vi "Send Next State.vi"(8 "error in (no error)":errorcluster, 9 "Data":variant, 10 "State":string, 11 "ExampleSimpleRootModel in":refnum<class "SimpleRootModel.lvclass">) -> (0 "error out":errorcluster, 3 "ExampleSimpleRootModel out":refnum<class "SimpleRootModel.lvclass">)   [LabVIEW 2018, in "MVAExamples.lvlib" / "SimpleRootModel.lvclass"]
uses:
  SimpleRootModel.lvclass
  <vilib>/ActorFramework/Actor/Actor.lvclass
  ExampleSimpleRootModel Messages/Execute State Msg/Execute State Msg.lvclass
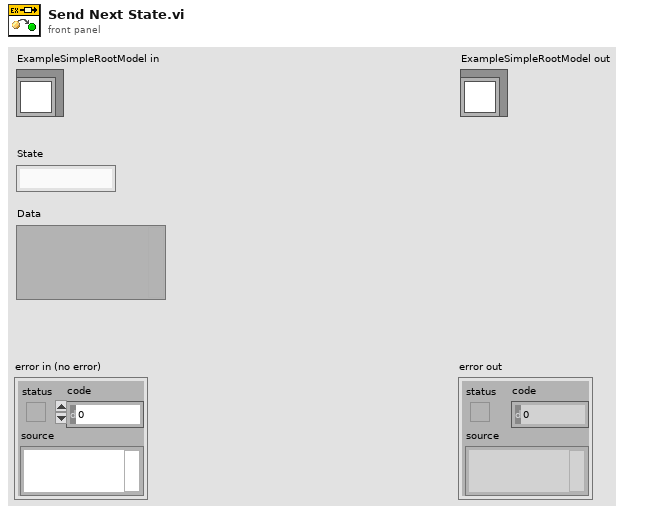
[diagram p1: front panel]
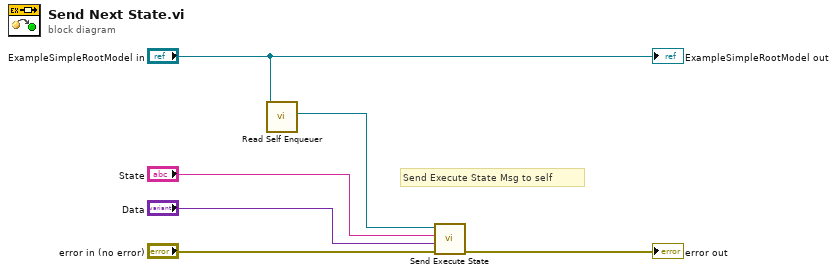
[diagram p0: block diagram]
diagram:
  # "Send Execute State Msg to self"
  n1 = call <vilib>:"Read Self Enqueuer.vi"("Actor"="ExampleSimpleRootModel in") -> ("Self Enqueuer"=w5:refnum<class "Message Enqueuer.lvclass">)  [unwired: 10 in]
  n2 = call "Send Execute State.vi"("error in (no error)"="error in (no error)", "Data"="Data", "State"="State", "Message Enqueuer"=w5) -> ("error out"=→"error out":errorcluster)  [unwired: 6 in, 1 out]
  "ExampleSimpleRootModel out" <- "ExampleSimpleRootModel in"
